vi "Read single image.vi"(8 "error in (no error)":errorcluster, 11 "data_loder_single_image in":refnum<class "data_loader_single_image.lvclass">) -> (0 "error out":errorcluster, 2 "Image":T1(plugin-control), 3 "data_loder_single_image out":refnum<class "data_loader_single_image.lvclass">)   [LabVIEW 2017, in "data_loader_single_image.lvclass"]
uses:
  data_loader_single_image.lvclass
  data_loader_single_image.lvclass/data_loader_single_image.ctl
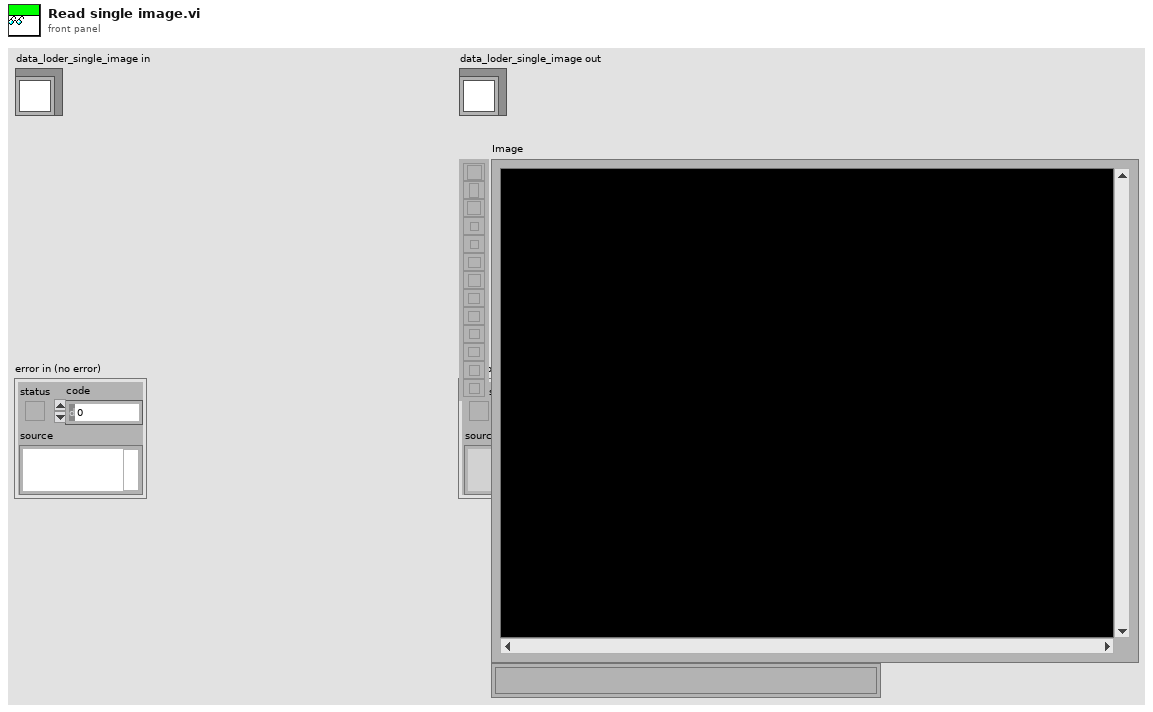
[diagram p1: front panel]
types:
  T1 = typedef "IMAQ Image.ctl" = refnum<image>
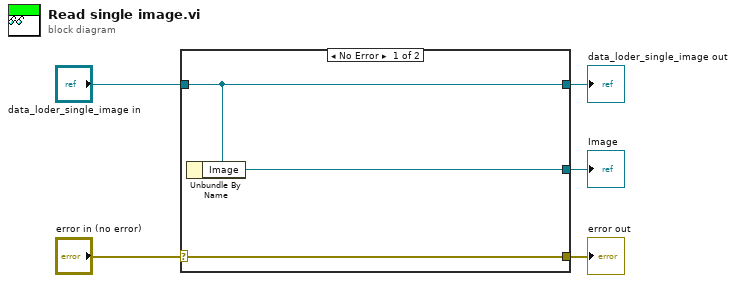
[diagram p0: block diagram]
diagram:
  n1 = case shown="No Error" "error in (no error)" {
    selector: "error in (no error)" -> [w8 w9]
    tunnel: [w8 w9] -> w4
    tunnel: [w7 w10] -> w2
    tunnel: "data_loder_single_image in" -> [w7 w10]
    tunnel: [w6 _] -> w1
    frame No Error {
      n2 = Unbundle By Name(w7) -> ("Image"=w6:T1)
    }
    frame Error {
    }
  }
  "error out" <- w4
  "data_loder_single_image out" <- w2
  "Image" <- w1
